vi "Limelight_Differential.vi"() -> (0 "DriveCommand":dbl(knob)=-0.0 scale=0.0..1.0, 1 "SteerCommand":dbl(knob)=nan scale=-1.0..1.0, 3 "TargetValid":bool)   [LabVIEW 2020]
uses:
  <vilib>/Rock Robotics/Network Tables/NT Read Number.vi
panel:
  in  "MaxDrive":dbl(slide)=0.6824817518248175 min=0.0 max=1.0 step=0.01 scale=0.0..1.0
  in  "DriveK":dbl(slide)=0.26277372262773724 min=0.0 max=1.0 step=0.05 scale=0.0..1.0
  in  "Limelight Goal Area":dbl(slide)=14.872262773722628 min=0.1 max=25.0 step=0.25 scale=0.0..25.0
  in  "AimDeadband":dbl min=0.0 max=10.0 step=0.25
  in  "MinSteerCommand":dbl(slide)=0.2717391304347826 min=0.0 max=0.5 step=0.05 scale=0.0..0.5
  in  "SteeringK":dbl(slide)=0.025362318840579712 min=0.0 max=0.25 step=0.01 scale=0.0..0.25
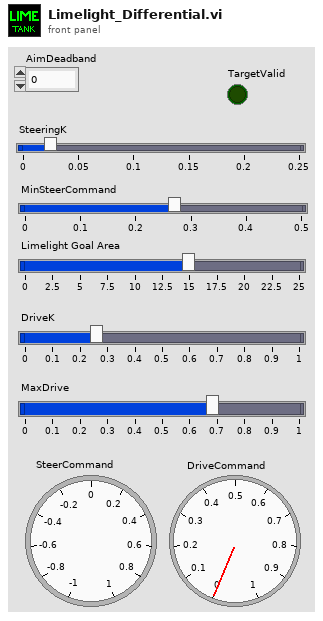
[diagram p1: front panel]
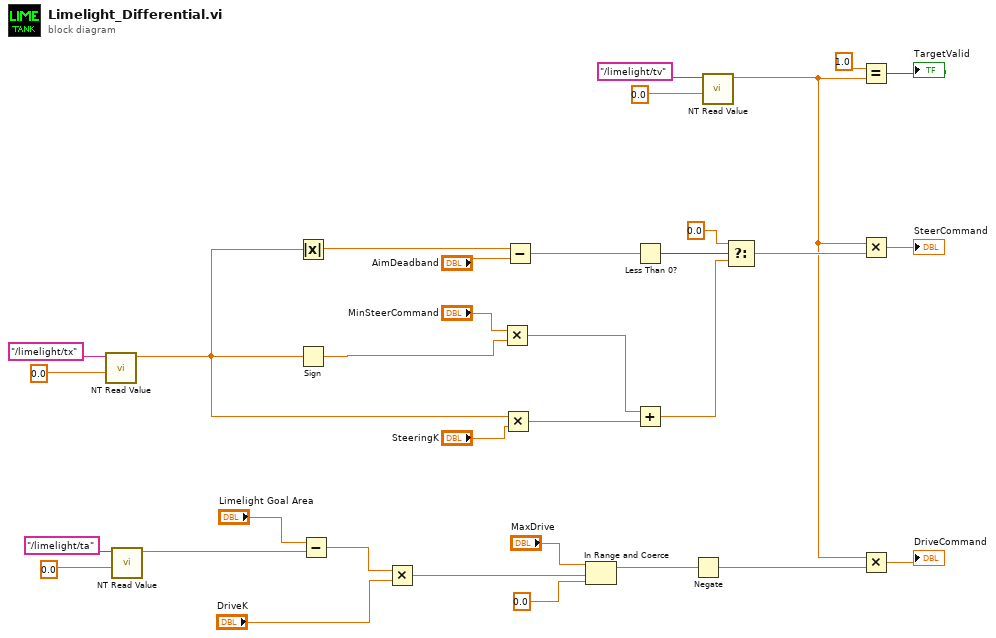
[diagram p0: block diagram]
diagram:
  n1 = call-poly <vilib>:"NT Read Value.vi"("Default Value"=0.0, "Name"="/limelight/tx") -> ("Numeric"=w5:dbl)  [unwired: 8 in, 1 out]
  n2 = call-poly <vilib>:"NT Read Value.vi"("Default Value"=0.0, "Name"="/limelight/ta") -> ("Numeric"=w14:dbl)  [unwired: 8 in, 1 out]
  n3 = Absolute Value(x=w5) -> (abs(x)=w29:dbl)
  n4 = Sign(1:w5) -> (0:w16:dbl)
  n5 = Subtract(x="Limelight Goal Area", y=w14) -> (x-y=w12:dbl)
  n6 = Multiply(x=w12, y="DriveK") -> (x*y=w11:dbl)
  n7 = Multiply(x="MinSteerCommand", y=w16) -> (x*y=w28:dbl)
  n8 = Multiply(x=w5, y="SteeringK") -> (x*y=w26:dbl)
  n9 = Subtract(x=w29, y="AimDeadband") -> (x-y=w31:dbl)
  n10 = In Range and Coerce(upper limit="MaxDrive", x=w11, lower limit=0.0) -> (coerced(x)=w7:dbl)  [unwired: 1 out]
  n11 = Less Than 0?(x=w31) -> (x < 0?=w32:bool)
  n12 = Add(x=w28, y=w26) -> (x+y=w4:dbl)
  n13 = Negate(x=w7) -> (-x=w6:dbl)
  n14 = call-poly <vilib>:"NT Read Value.vi"("Default Value"=0.0, "Name"="/limelight/tv") -> ("Numeric"=w3:dbl)  [unwired: 8 in, 1 out]
  n15 = Select(t=0.0, s=w32, f=w4) -> (s? t:f=w19:dbl)
  n16 = Equal?(x=1.0, y=w3) -> (x = y?=→"TargetValid":bool)
  n17 = Multiply(x=w3, y=w19) -> (x*y=→"SteerCommand":dbl)
  n18 = Multiply(x=w3, y=w6) -> (x*y=→"DriveCommand":dbl)
